vi "test Deployment No RaF CD.vi"(8 "error in (no error)":errorcluster, 11 "TestCase in":refnum<class "Routing and Faulting System Tests.lvclass">) -> (0 "error out":errorcluster, 3 "TestCase out":refnum<class "Routing and Faulting System Tests.lvclass">)   [LabVIEW 2017, in "Routing and Faulting System Tests.lvclass"]
uses:
  Routing and Faulting System Tests.lvclass
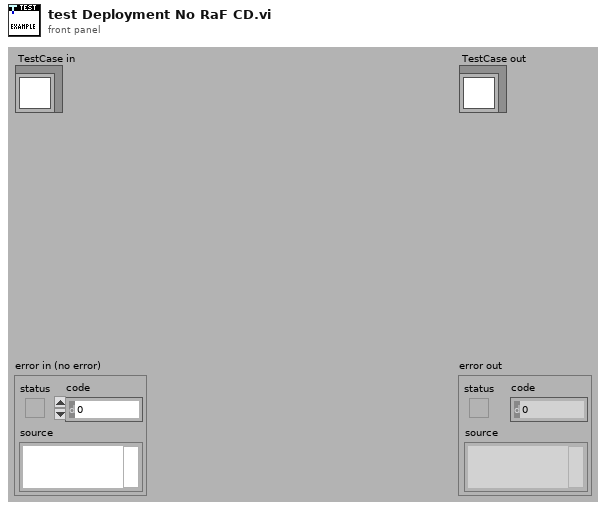
[diagram p1: front panel]
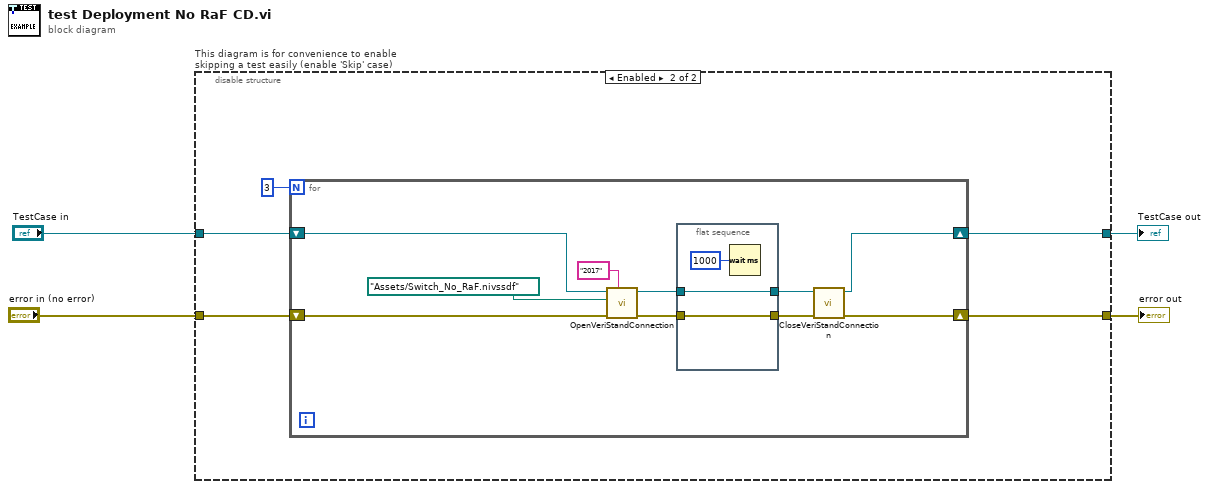
[diagram p0: block diagram]
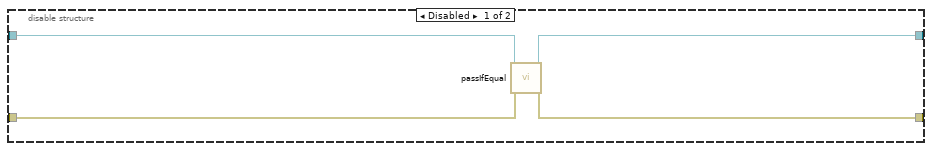
[diagram p2: hidden frame]
diagram:
  n1 = disable-structure "This diagram is for convenience to enable skipping a test easily (enable 'Skip' case)" shown="Enabled" {
    disable-tunnel: "TestCase in" -> [w8 w13]
    disable-tunnel: [w7 w10] -> w1
    disable-tunnel: [w6 w9] -> w3
    disable-tunnel: "error in (no error)" -> [w5 w12]
    frame Disabled {
      n2 = call-dynamic "passIfEqual.vi"("error in (no error)"=w5, "TestCase in"=w8) -> ("error out"=w6:errorcluster, "TestCase out"=w7:refnum<class "Routing and Faulting System Tests.lvclass">)  [unwired: 8 in]
    }
    frame Enabled {
      n3 = for {
        N: 3 -> [_]
        shift-right: [w19] -> w10
        shift-left: w13 -> [w21]
        shift-right: [w18] -> w9
        shift-left: w12 -> [w20]
        n4 = call-dynamic "OpenVeriStandConnection.vi"("Minimum VeriStand Version (2015)"="2017", "error in (no error)"=w20, "System Definition File"=path "Assets/Switch_No_RaF.nivssdf", "VeriStand Test Case in"=w21) -> ("error out"=w16:errorcluster, "VeriStand Test Case out"=w17:refnum<class "Routing and Faulting System Tests.lvclass">)  [unwired: 5 in, 1 out]
        n5 = flat-sequence {
          tunnel: w17 -> [w26]
          tunnel: w16 -> [w25]
          tunnel: [w26] -> w15
          tunnel: [w25] -> w14
          frame #0 {
            n6 = Wait (ms)(milliseconds to wait=u32 1000) -> ()  [unwired: 1 out]
          }
        }
        n7 = call-dynamic "CloseVeriStandConnection.vi"("error in (no error)"=w14, "VeriStand Test Case in"=w15) -> ("error out"=w18:errorcluster, "VeriStand Test Case out"=w19:refnum<class "Routing and Faulting System Tests.lvclass">)  [unwired: 8 in]
      }
    }
  }
  "error out" <- w3
  "TestCase out" <- w1
